vi "LowIF_audiojack_exe.vi"() -> ()   [LabVIEW 2015]
doc: "This example demonstrates how to use the Short-time Fourier Transform (STFT Spectrograms) VI to analyze the Time-Frequency spectrogram."
uses:
  <vilib>/sound2/lvsound2.llb/Sampling Mode.ctl
  <vilib>/Analysis/3filter.llb/Filter Passband Type.ctl
  <vilib>/Analysis/2dsp.llb/Complex FFT.vi
  <vilib>/sound2/lvsound2.llb/Sound Input Read (DBL).vi
  <vilib>/Analysis/3filter.llb/Chebyshev Filter (DBL).vi
  <vilib>/Analysis/baseanly.llb/Mean (CDB).vi
  <vilib>/Analysis/NI_AALPro.lvlib
  <vilib>/Analysis/NI_AALBase.lvlib
  <vilib>/Analysis/NI_AAL_SigProc.lvlib
panel:
  out "Heart rate":dbl format="%#.0f"
  out "Respiration rate":dbl format="%#.0f"
  in  "Minimun dB":dbl=-15.0 max=0.0
  in  "Frequency Range":dbl(slide)=3.2 caption="Beats per Min (x60)" min=1.0 step=0.1 scale=0.0..160.0
  out "Frequency":dbl[](graph) caption="I/Q Signal"
  in  "bits per sample":i32=16
  in  "number of channels":i32=2
  in  "sample rate (S/s)":dbl=320.0
  in  "data length":i32=4800
  out "I/Q Signal":dynamicdata(graph)
  in  "number of samples/ch":i32=32
  in  "device ID":u32
  in  "Stop":bool
  # "Low-IF interferometry radar data processing"
  # "Version: 2\nZhengyu Peng\nC. Li Lab\nTexas Tech University\nSep. 2015"
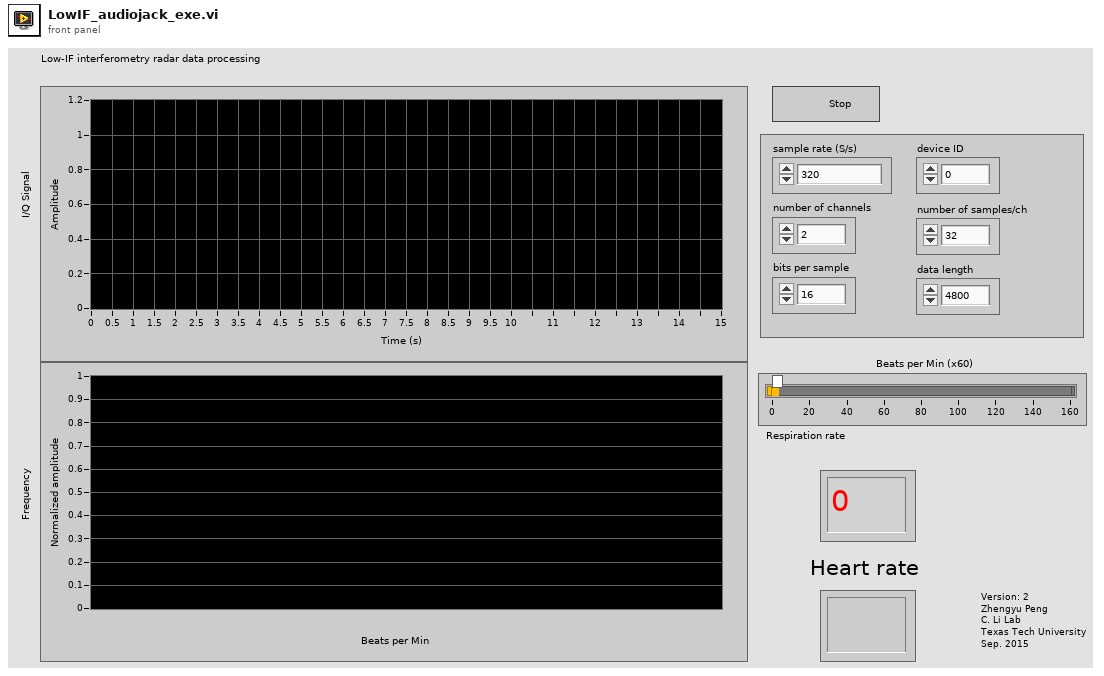
[diagram p1: front panel]
types:
  T1 = typedef "Sampling Mode.ctl" = i32
  T2 = cluster{"sample rate (S/s)":dbl, "number of channels":i32, "bits per sample ":i32}
  T3 = typedef "Sound Input Task ID.ctl" = u32
  T4 = typedef "NI_AALBase.lvlib/Filter Passband Type.ctl" = enum32{"Lowpass", "Highpass", "Bandpass", "Bandstop"}
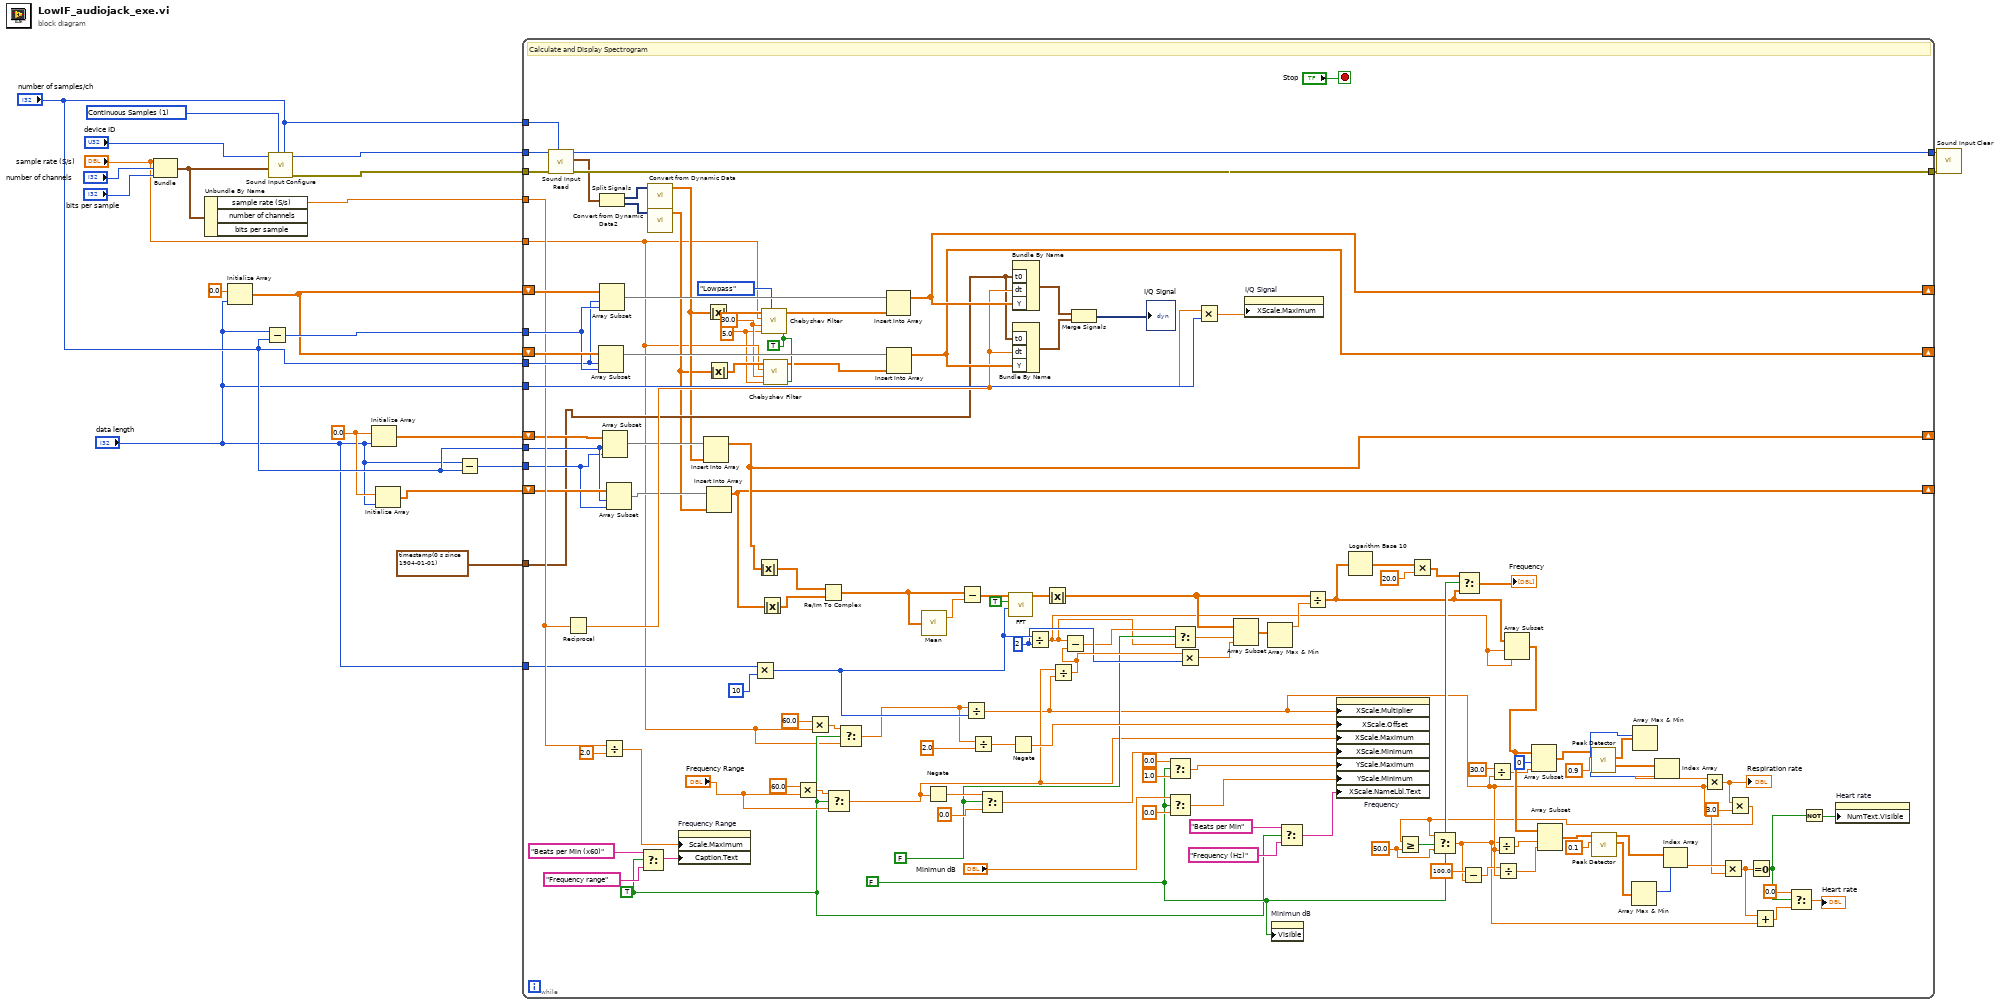
[diagram p0: block diagram]
diagram:
  w3 = T1 1 items=["Finite Samples", "Continuous Samples"] ("sample mode")
  w6 = 0.0 ("element")
  n1 = Bundle("sample rate (S/s)"="sample rate (S/s)", "number of channels"="number of channels", "bits per sample"="bits per sample") -> (w10:T2)  [unwired: 1 in]
  n2 = Unbundle By Name(w10) -> ("sample rate (S/s)"=w13:dbl)  [unwired: 2 out]
  n3 = Initialize Array(0.0 ("element"), "data length") -> (w14:dbl[])
  n4 = Subtract(x="data length", y="number of samples/ch") -> (x-y=w15:i32)
  n5 = call <vilib>:"Sound Input Configure.vi"("number of samples/ch"="number of samples/ch", "sample mode"=w3, "sound format"=w10, "device ID"="device ID") -> ("error out"=w19:errorcluster, "task ID"=w20:T3)  [unwired: 6 in]
  n6 = Initialize Array(w6, "data length") -> (w9:dbl[])
  n7 = Initialize Array(w6, "data length") -> (w5:dbl[])
  n8 = Subtract(x="data length", y="number of samples/ch") -> (x-y=w8:i32)
  n9 = while {
    tunnel: w20 -> [w151]
    tunnel: "number of samples/ch" -> [w150]
    tunnel: w19 -> [w149]
    tunnel: [w148] -> w18
    tunnel: [w147] -> w17
    shift-right: [w131] -> _
    shift-left: w14 -> [w143]
    tunnel: w15 -> [w140]
    shift-right: [w130] -> _
    shift-left: w14 -> [w141]
    tunnel: "number of samples/ch" -> [w137]
    tunnel: w13 -> [w133]
    tunnel: "data length" -> [w135]
    tunnel: "data length" -> [w116]
    tunnel: "sample rate (S/s)" -> [w49]
    shift-right: [w72] -> _
    shift-left: w9 -> [w122]
    tunnel: w8 -> [w118]
    tunnel: "number of samples/ch" -> [w119]
    shift-right: [w70] -> _
    shift-left: w5 -> [w120]
    tunnel: timestamp(0 s since 1904-01-01) ("t0") -> [w113]
    stop <- "Stop" stop-if-true
    w22 = 50.0 ("y")
    w48 = 30.0 ("high cutoff freq: fh")
    w46 = TRUE ("init/cont (init:F)")
    w47 = 5.0 ("high cutoff freq: fh")
    w99 = FALSE ("negative frequency?")
    w89 = FALSE ("dB scale?")
    w76 = TRUE ("scale to beats per min?")
    w102 = 2 ("y")
    # "Calculate and Display Spectrogram"
    n10 = call-poly <vilib>:"Sound Input Read.vi"("number of samples/ch"=w150, "error in (no error)"=w149, "task ID"=w151) -> ("error out"=w147:errorcluster, "data"=w144:waveform(dbl)[], "task ID out"=w148:T3)  [unwired: 6 in]
    n11 = Reciprocal(x=w133) -> (1/x=w126:dbl)
    n12 = Array Subset(array=w141, index=w137, length=w140) -> (w139:dbl[])
    n13 = Split Signals(w144) -> (w146:dynamicdata, w145:dynamicdata)  [unwired: 2 out]
    n14 = Array Subset(array=w143, index=w137, length=w140) -> (w142:dbl[])
    n15 = Divide(x=w133, y=2.0) -> (x/y=w112:dbl)
    n16 = Array Subset(array=w122, index=w119, length=w118) -> (w121:dbl[])
    n17 = Array Subset(array=w120, index=w119, length=w118) -> (w117:dbl[])
    n18 = Select(t="Beats per Min (x60)" ("X Scale.Name Label.Text"), s=w76, f="Frequency range" ("X Scale.Name Label.Text")) -> (s? t:f=w75:string)
    n19 = call "Convert from Dynamic Data"("Dynamic Data Type"=w146) -> ("Array"=w55:dbl[])  [unwired: 3 out]
    n20 = call "Convert from Dynamic Data2"("Dynamic Data Type"=w145) -> ("Array"=w51:dbl[])  [unwired: 3 out]
    n21 = property on="Frequency Range" class="Slide (strict)"("Scale.Maximum"=w112, "Caption.Text"=w75) -> ()  [unwired: 2 in, 2 out]
    n22 = Insert Into Array(array=w121, new element=w55) -> (w72:dbl[])  [unwired: 1 in]
    n23 = Absolute Value(x=w55) -> (abs(x)=w54:dbl[])
    n24 = Absolute Value(x=w51) -> (abs(x)=w50:dbl[])
    n25 = Insert Into Array(array=w117, new element=w51) -> (w70:dbl[])  [unwired: 1 in]
    n26 = Multiply(x=w116, y=10) -> (x*y=w105:i32)
    n27 = Absolute Value(x=w72) -> (abs(x)=w71:dbl[])
    n28 = Absolute Value(x=w70) -> (abs(x)=w69:dbl[])
    n29 = call-poly <vilib>:"Chebyshev Filter.vi"("init/cont (init:F)"=w46, "filter type"=Filter_Passband_Type."Lowpass", "low cutoff freq: fl"=w47, "high cutoff freq: fh"=w48, "sampling freq: fs"=w49, "X"=w54) -> ("Filtered X"=w52:dbl[])  [unwired: 4 in, 1 out]
    n30 = call-poly <vilib>:"Chebyshev Filter.vi"("init/cont (init:F)"=w46, "low cutoff freq: fl"=w47, "high cutoff freq: fh"=w48, "sampling freq: fs"=w49, "X"=w50) -> ("Filtered X"=w45:dbl[])  [unwired: 5 in, 1 out]
    n31 = Multiply(x=60.0, y="Frequency Range") -> (x*y=w81:dbl)
    n32 = Multiply(x=60.0, y=w49) -> (x*y=w84:dbl)
    n33 = Re/Im To Complex(1:w69, 2:w71) -> (0:w73:cdb[])
    n34 = Select(t=w81, s=w76, f="Frequency Range") -> (s? t:f=w80:dbl)
    n35 = Select(t=w84, s=w76, f=w49) -> (s? t:f=w83:dbl)
    n36 = Insert Into Array(array=w142, new element=w52) -> (w131:dbl[])  [unwired: 1 in]
    n37 = Insert Into Array(array=w139, new element=w45) -> (w130:dbl[])  [unwired: 1 in]
    n38 = call-poly <vilib>:"Mean.vi"("X"=w73) -> ("mean"=w129:cdb)  [unwired: 1 out]
    n39 = Negate(x=w80) -> (-x=w109:dbl)
    n40 = Subtract(x=w73, y=w129) -> (x-y=w114:cdb[])
    n41 = Divide(x=w83, y=w105) -> (x/y=w34:dbl)
    n42 = Divide(x=w83, y=2.0) -> (x/y=w124:dbl)
    n43 = Select(t=w109, s=w99, f=0.0) -> (s? t:f=w111:dbl)
    n44 = call-poly <vilib>:"FFT.vi"("FFT size"=w105, "shift?"=TRUE, "X"=w114) -> ("FFT {X}"=w127:cdb[])  [unwired: 7 in, 1 out]
    n45 = Negate(x=w124) -> (-x=w123:dbl)
    n46 = Bundle By Name("t0"=w113, "dt"=w126, "Y"=w131) -> (w138:waveform(dbl))  [unwired: 1 out]
    n47 = Bundle By Name("t0"=w113, "dt"=w126, "Y"=w130) -> (w136:waveform(dbl))  [unwired: 1 out]
    n48 = Divide(x=w105, y=w102) -> (x/y=w30:dbl)
    n49 = Absolute Value(x=w127) -> (abs(x)=w108:dbl[])
    n50 = Divide(x=w80, y=w34) -> (x/y=w103:dbl)
    n51 = Subtract(x=w30, y=w103) -> (x-y=w100:dbl)
    n52 = Merge Signals(w138, w136) -> (→"I/Q Signal":dynamicdata)
    n53 = Select(t=0.0, s=w89, f=1.0) -> (s? t:f=w91:dbl)
    n54 = Select(t="Minimun dB", s=w89, f=0.0) -> (s? t:f=w95:dbl)
    n55 = Select(t=w100, s=w99, f=w30) -> (s? t:f=w101:dbl)
    n56 = Multiply(x=w103, y=w102) -> (x*y=w104:dbl)
    n57 = Multiply(x=w126, y=w135) -> (x*y=w134:dbl)
    n58 = Array Subset(array=w108, index=w101, length=w104) -> (w107:dbl[])
    n59 = property on="I/Q Signal" class="WFGraph (strict)"("XScale.Maximum"=w134) -> ()  [unwired: 2 in, 2 out]
    n60 = Array Max & Min(array=w107) -> (max value=w106:dbl)  [unwired: 3 out]
    n61 = property on="Minimun dB" class="DigNum (strict)"("Visible"=w89) -> ()  [unwired: 2 in, 2 out]
    n62 = Select(t="Beats per Min" ("X Scale.Name Label.Text"), s=w76, f="Frequency (Hz)" ("X Scale.Name Label.Text")) -> (s? t:f=w87:string)
    n63 = Divide(x=w108, y=w106) -> (x/y=w59:dbl[])
    n64 = property on="Frequency" class="WFGraph (strict)"("XScale.Multiplier"=w34, "XScale.Offset"=w123, "XScale.Maximum"=w80, "XScale.Minimum"=w111, "YScale.Maximum"=w91, "YScale.Minimum"=w95, "XScale.NameLbl.Text"=w87) -> ()  [unwired: 2 in, 2 out]
    n65 = Logarithm Base 10(1:w59) -> (0:w98:dbl[])
    n66 = Multiply(x=w98, y=20.0) -> (x*y=w67:dbl[])
    n67 = Select(t=w67, s=w89, f=w59) -> (s? t:f=→"Frequency":dbl[])
    n68 = Divide(x=30.0, y=w34) -> (x/y=w36:dbl)
    n69 = Array Subset(array=w59, index=w30, length=w30) -> (w38:dbl[])
    n70 = Array Subset(array=w38, index=0, length=w36) -> (w39:dbl[])
    n71 = call <vilib>:"Peak Detector.vi"("threshold"=0.9, "X"=w39) -> ("Amplitudes"=w43:dbl[], "Locations"=w44:dbl[])  [unwired: 5 in, 3 out]
    n72 = Array Max & Min(array=w43) -> (max index (indices)=w42:i32)  [unwired: 3 out]
    n73 = Index Array(array=w44, index=w42) -> (element=w66:dbl)
    n74 = Multiply(x=w66, y=w34) -> (x*y=w29:dbl)
    "Respiration rate" <- w29
    n75 = Multiply(x=w29, y=3.0) -> (x*y=w24:dbl)
    n76 = Greater Or Equal?(x=w24, y=w22) -> (x >= y?=w25:bool)
    n77 = Select(t=w24, s=w25, f=w22) -> (s? t:f=w23:dbl)
    n78 = Subtract(x=100.0, y=w23) -> (x-y=w26:dbl)
    n79 = Divide(x=w23, y=w34) -> (x/y=w65:dbl)
    n80 = Divide(x=w26, y=w34) -> (x/y=w64:dbl)
    n81 = Array Subset(array=w38, index=w65, length=w64) -> (w63:dbl[])
    n82 = call <vilib>:"Peak Detector.vi"("threshold"=0.1, "X"=w63) -> ("Amplitudes"=w41:dbl[], "Locations"=w61:dbl[])  [unwired: 5 in, 3 out]
    n83 = Array Max & Min(array=w41) -> (max index (indices)=w40:i32)  [unwired: 3 out]
    n84 = Index Array(array=w61, index=w40) -> (element=w60:dbl)
    n85 = Multiply(x=w60, y=w34) -> (x*y=w57:dbl)
    n86 = Equal To 0?(x=w57) -> (x = 0?=w32:bool)
    n87 = Add(x=w57, y=w23) -> (x+y=w58:dbl)
    n88 = Select(t=0.0, s=w32, f=w58) -> (s? t:f=→"Heart rate":dbl)
    n89 = Not(x=w32) -> (.not. x?=w31:bool)
    n90 = property on="Heart rate" class="DigNum (strict)"("NumText.Visible"=w31) -> ()  [unwired: 2 in, 2 out]
  }
  n91 = call <vilib>:"Sound Input Clear.vi"("error in (no error)"=w17, "task ID"=w18) -> ()  [unwired: 9 in, 1 out]
